vi "Create.vi"(7 ".NET Process in":refnum<class ".NET Process.lvclass">, 8 "error in (no error)":errorcluster, 9 "Working Directory (App Directory)":path, 10 "Arguments (empty)":string, 11 "Process File Name":string) -> (0 "error out":errorcluster, 2 "Public Events":T1, 3 ".NET Process out":refnum<class ".NET Process.lvclass">)   [LabVIEW 2019, in ".NET Process.lvclass"]
uses:
  .NET Process.lvclass
  .NET Process.lvclass/.NET Process.ctl
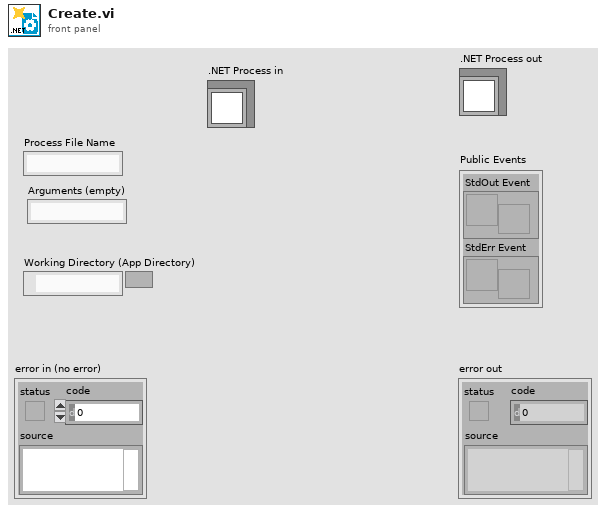
[diagram p1: front panel]
types:
  T1 = cluster{"StdOut Event":refnum<user-event>, "StdErr Event":refnum<user-event>}
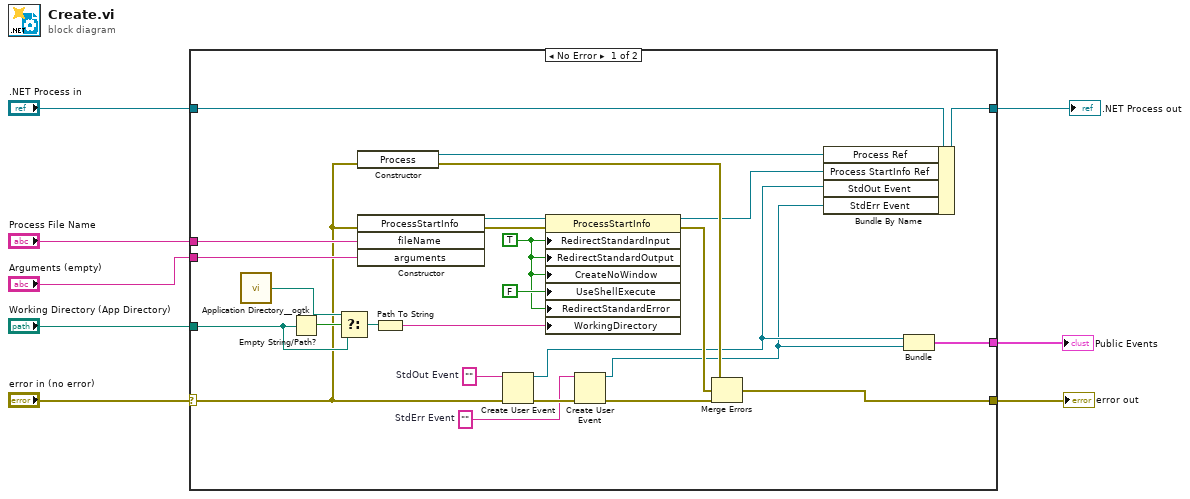
[diagram p0: block diagram]
diagram:
  n1 = case shown="No Error" "error in (no error)" {
    selector: "error in (no error)" -> [w12 w36]
    tunnel: [w22 w36] -> w7
    tunnel: [w21 w35] -> w5
    tunnel: ".NET Process in" -> [w20 w35]
    tunnel: "Process File Name" -> [w28 _]
    tunnel: "Arguments (empty)" -> [w27 _]
    tunnel: "Working Directory (App Directory)" -> [w24 _]
    tunnel: [w11 _] -> w1
    frame No Error {
      w14 = ""  # StdErr Event
      w16 = ""  # StdOut Event
      w31 = TRUE ("RedirectStandardInput")
      n2 = call "Application Directory__ogtk.vi"() -> ("Application Directory (+ Relative)"=w17:path)  [unwired: 1 in]
      n3 = Empty String/Path?(string/path=w24) -> (empty?=w25:bool)
      n4 = Select(t=w17, s=w25, f=w24) -> (s? t:f=w23:path)
      n5 = constructor class="Process"(error in=w12) -> (reference out=w19:refnum<k24>, error out=w30:errorcluster)  [unwired: 2 in, 1 out]
      n6 = constructor class="ProcessStartInfo"(error in=w12, "fileName"=w28, "arguments"=w27) -> (reference out=w33:refnum<k24>, error out=w34:errorcluster)  [unwired: 2 in, 3 out]
      n7 = Path To String(path=w23) -> (string=w26:string)
      n8 = Create User Event(user event datatype=w16, error in=w12) -> (user event=w10:refnum<user-event>, error out=w15:errorcluster)
      n9 = property class="ProcessStartInfo"(reference=w33, error in=w34, "RedirectStandardInput"=w31, "RedirectStandardOutput"=w31, "CreateNoWindow"=w31, "UseShellExecute"=FALSE, "RedirectStandardError"=w31, "WorkingDirectory"=w26) -> (reference out=w18:refnum<k24>, error out=w29:errorcluster)
      n10 = Create User Event(user event datatype=w14, error in=w15) -> (user event=w9:refnum<user-event>, error out=w13:errorcluster)
      n11 = Merge Errors(w30, w29, w13) -> (w22:errorcluster)
      n12 = Bundle By Name(cluster=w20, "Process Ref"=w19, "Process StartInfo Ref"=w18, "StdOut Event"=w10, "StdErr Event"=w9) -> (w21:refnum<class ".NET Process.lvclass">)
      n13 = Bundle("StdOut Event"=w10, "StdErr Event"=w9) -> (w11:T1)  [unwired: 1 in]
    }
    frame Error {
    }
  }
  "error out" <- w7
  ".NET Process out" <- w5
  "Public Events" <- w1
